vi "Analog Read.vi"() -> ()   [LabVIEW 2018]
uses:
  <vilib>/NI/Modbus Library/API/Wrapper/Create Serial Master.vi
  <vilib>/NI/Modbus Library/API/Master/Modbus Master.lvclass
  <vilib>/NI/Modbus Library/API/Wrapper/API Main.lvlib
  <vilib>/ptbypt/NI_PtbyPt.lvlib
panel:
  out "Date Time":string
  out "LED 2":bool
  out "LED 1":bool
  out "LED 2":u16
  out "LED 1":u16
  out "Sensor 2":dbl
  out "Sensor 1":dbl
  out "Read register values":u16[](array[numeric])
  in  "USB Serial Port":refnum<visa-resource-name>
  out "Waveform Chart":dynamicdata(graph)
  out "Table":string[][](table)
  in  "Home Button":bool=TRUE
  in  "Stop":bool
  out "Result":string
  in  "Play Button":bool=TRUE
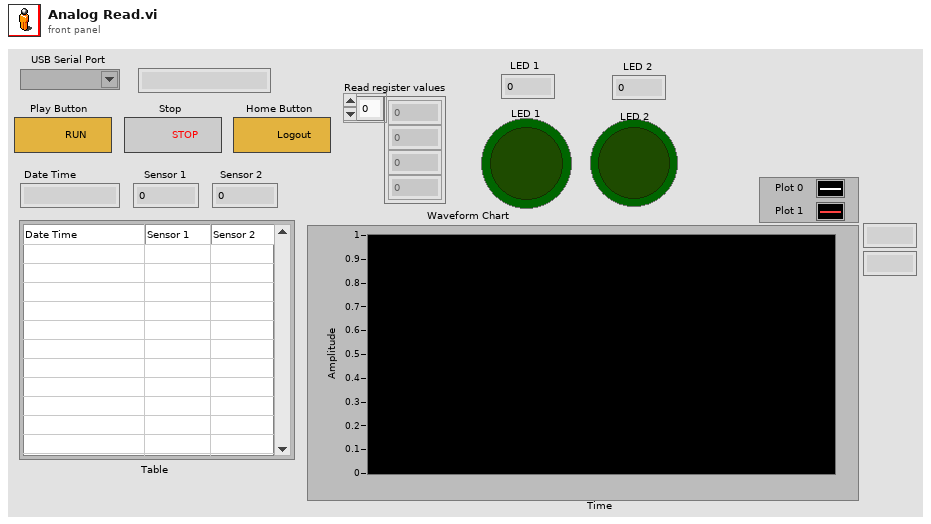
[diagram p1: front panel]
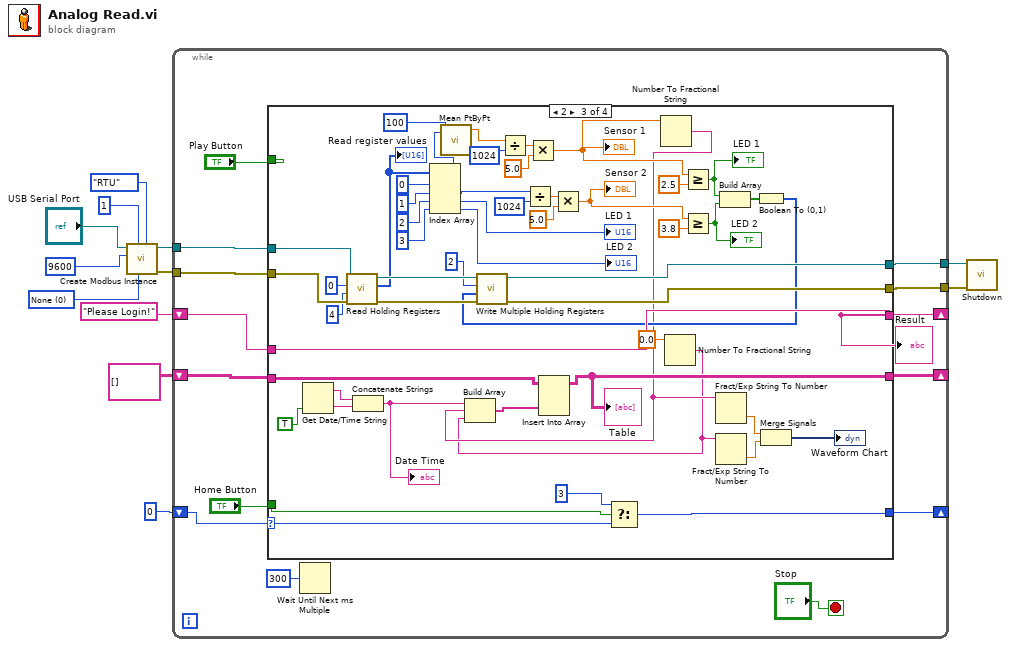
[diagram p0: block diagram]
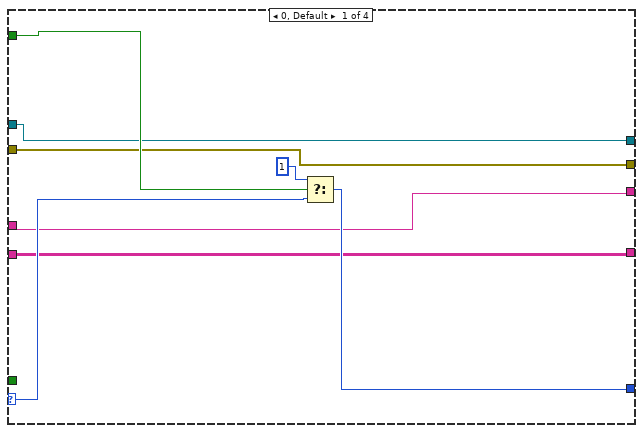
[diagram p2: hidden frame]
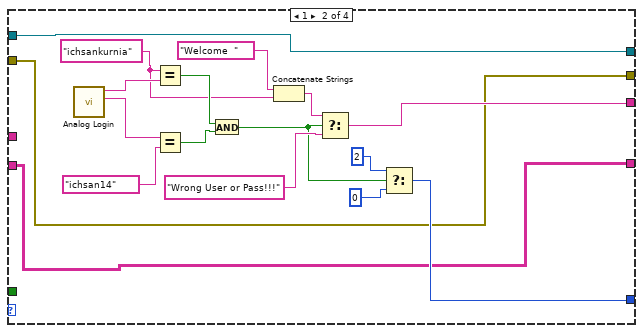
[diagram p3: hidden frame]
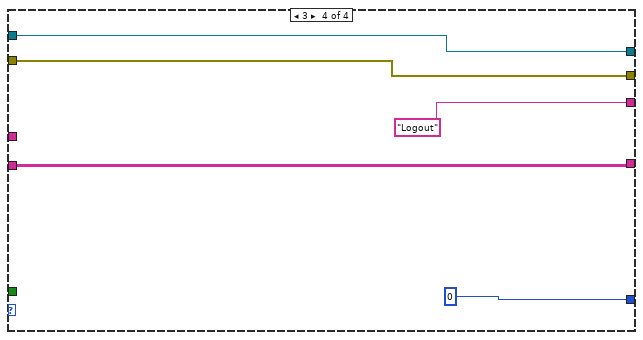
[diagram p4: hidden frame]
diagram:
  w7 = u16 0 items=["None", "Odd", "Even", "Mark", "Space"] ("parity (even)")
  n1 = call-poly <vilib>:"Create Modbus Instance.vi"("serial type"=enum16{"RTU", "ASCII"}."RTU", "parity (even)"=w7, "unit ID"=u8 1, "baud rate"=u32 9600 ("byte count"), "VISA resource name"="USB Serial Port") -> ("error out"=w4:errorcluster, "serial master instance"=w3:refnum<class "Modbus Master.lvclass">)  [unwired: 5 in]
  n2 = while {
    shift-right: [w26] -> _
    shift-left: 0 -> [w22]
    shift-right: [w21] -> _
    shift-left: "Please Login!" ("String") -> [w20]
    tunnel: w3 -> [w19]
    tunnel: w4 -> [w18]
    tunnel: [w17] -> w2
    tunnel: [w16] -> w1
    shift-right: [w14] -> _
    shift-left: string[][] [] -> [w13]
    stop <- "Stop" stop-if-true
    n3 = case shown="2" w22 {
      selector: w22 -> [w32 _ w101 _]
      tunnel: [w34 w51 w103 0] -> w26
      tunnel: "Play Button" -> [w33 _ _ _]
      tunnel: "Home Button" -> [_ _ w100 _]
      tunnel: [w30 w41 w99 "Logout" ("String")] -> w21
      tunnel: w20 -> [w30 _ w99 _]
      tunnel: w19 -> [w29 w38 w91 w106]
      tunnel: w18 -> [w28 w37 w90 w105]
      tunnel: [w28 w37 w86 w105] -> w17
      tunnel: [w29 w38 w87 w106] -> w16
      tunnel: [w27 w36 w94 w104] -> w14
      tunnel: w13 -> [w27 w36 w95 w104]
      frame 0, Default {
        n4 = Select(t=1, s=w33, f=w32) -> (s? t:f=w34:i32)
      }
      frame 1 {
        w35 = "ichsankurnia"
        n5 = call "Analog Login.vi"() -> ("Password 2"=w39:string, "User Name 2"=w40:string)  [unwired: 9 in, 1 out]
        n6 = Equal?(x=w35, y=w40) -> (x = y?=w44:bool)
        n7 = Equal?(x=w39, y="ichsan14") -> (x = y?=w43:bool)
        n8 = And(x=w44, y=w43) -> (x .and. y?=w45:bool)
        n9 = Concatenate Strings("Welcome  ", w35) -> (w48:string)
        n10 = Select(t=w48, s=w45, f="Wrong User or Pass!!!") -> (s? t:f=w41:string)
        n11 = Select(t=2, s=w45, f=0) -> (s? t:f=w51:i32)
      }
      frame 2 {
        n12 = Get Date/Time String(want seconds? (F)=TRUE) -> (date string=w97:string, time string=w96:string)  [unwired: 2 in]
        n13 = call-dynamic "Read Holding Registers.vi"("error in"=w90, "number of inputs"=u16 4, "starting address"=u16 0, "Modbus master in"=w91) -> ("error out"=w84:errorcluster, "register values"=w82:u16[], "Modbus master out"=w85:refnum<class "Modbus Master.lvclass">)  [unwired: 5 in]
        "Read register values" <- w82
        n14 = Concatenate Strings(w97, w96) -> (w93:string)
        "Date Time" <- w93
        n15 = Index Array(array=w82, index #1=0, index #2=1, index #3=2, index #4=3) -> (element #1=w55:u16, element #2=w71:u16, element #3=→"LED 1":u16, element #4=→"LED 2":u16)
        n16 = call <vilib>:"Mean PtByPt.vi"("x"=w55, "sample length"=100) -> ("mean"=w54:dbl)  [unwired: 2 in, 1 out]
        n17 = Divide(x=w54, y=u16 1024) -> (x/y=w76:dbl)
        n18 = Divide(x=w71, y=u16 1024) -> (x/y=w73:dbl)
        n19 = Multiply(x=w76, y=5.0) -> (x*y=w62:dbl)
        "Sensor 1" <- w62
        n20 = Multiply(x=w73, y=5.0) -> (x*y=w61:dbl)
        "Sensor 2" <- w61
        n21 = Select(t=3, s=w100, f=w101) -> (s? t:f=w103:i32)
        n22 = Number To Fractional String(number=w62) -> (F-format string=w60:string)  [unwired: 3 in]
        n23 = Number To Fractional String(number=0.0) -> (F-format string=w59:string)  [unwired: 3 in]
        n24 = Build Array(w93, w60, w59) -> (w92:string[])
        n25 = Insert Into Array(array=w95, new element=w92) -> (w94:string[][])  [unwired: 2 in]
        "Table" <- w94
        n26 = Greater Or Equal?(x=w62, y=2.5) -> (x >= y?=w66:bool)
        "LED 1" <- w66
        n27 = Greater Or Equal?(x=w61, y=3.8) -> (x >= y?=w63:bool)
        "LED 2" <- w63
        n28 = Fract/Exp String To Number(string=w60) -> (number=w58:dbl)  [unwired: 3 in, 1 out]
        n29 = Fract/Exp String To Number(string=w59) -> (number=w57:dbl)  [unwired: 3 in, 1 out]
        n30 = Build Array(w66, w63) -> (w65:bool[])
        n31 = Boolean To (0,1)(Boolean=w65) -> (0, 1=w64:i16[])
        n32 = call-dynamic "Write Multiple Holding Registers.vi"("error in"=w84, "registers to write"=w64, "starting address"=u16 2, "Modbus master in"=w85) -> ("error out"=w86:errorcluster, "Modbus master out"=w87:refnum<class "Modbus Master.lvclass">)  [unwired: 6 in]
        n33 = Merge Signals(w58, w57) -> (→"Waveform Chart":dynamicdata)
      }
      frame 3 {
      }
    }
    "Result" <- w21
    n34 = Wait Until Next ms Multiple(millisecond multiple=u32 300) -> ()  [unwired: 1 out]
  }
  n35 = call-dynamic "Shutdown.vi"("error in"=w2, "Modbus master in"=w1) -> ()  [unwired: 9 in, 1 out]
